vi "viBuildFrame.vi"(1 "input variable":u8[](array[numeric])) -> (0 "output bytes":u8[](array[numeric]))   [LabVIEW 2009]
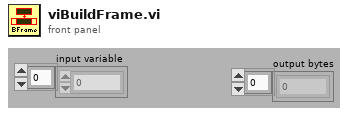
[diagram p1: front panel]
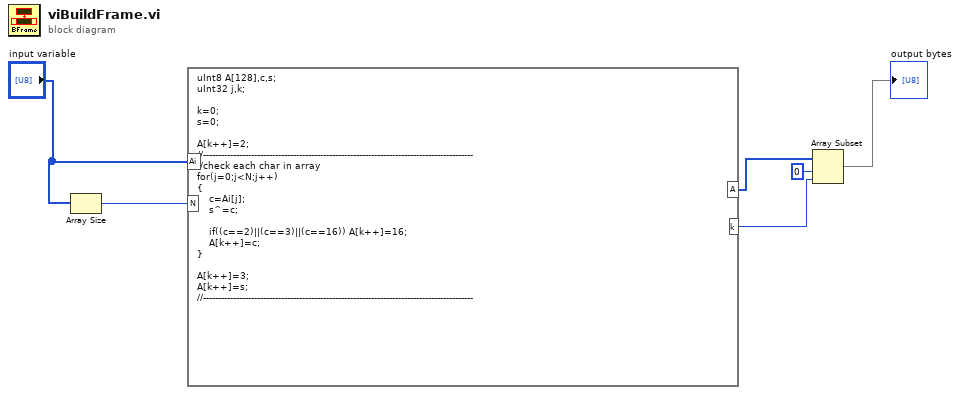
[diagram p0: block diagram]
diagram:
  n1 = Array Size(array="input variable") -> (size(s)=w6:i32)
  n2 = formula code="uInt8 A[128],c,s;\nuInt32 j,k;\n\nk=0;\ns=0;\n\nA[k++]=2;\n//------------------------------------------------------------------------------------------\n//check each char in array\nfor(j=0;j<N;j++)\n{\n    c=Ai[j];\n    s^=c;\n\n    if((c==2)||(c==3)||(c==16)) A[k++]=16;\n    A[k++]=c;    \n}\n\nA[k++]=3;\nA[k++]=s;\n//------------------------------------------------------------------------------------------"("Ai"="input variable", "N"=w6) -> ("k"=w2:u32, "A"=w4:u8[])
  n3 = Array Subset(array=w4, index=0, length=w2) -> (→"output bytes":u8[])
